vi "Sweep iteration instruction generator (SubVI).vi"(4 "Current iteration":i32, 6 "Angle theta [degrees]":dbl, 7 "Sweep plane & fixed axis":string, 9 "Magnetic field strength [µT]":dbl, 10 "Number of steps":dbl, 11 "Octant":string) -> (0 "Magnetic field z [µT]":dbl, 1 "Magnetic field y [µT]":dbl, 2 "Magnetic field x [µT]":dbl, 3 "Azimuthal angle \"phi\"":dbl, 5 "String: instructions to be sent to PS":string)   [LabVIEW 2018]
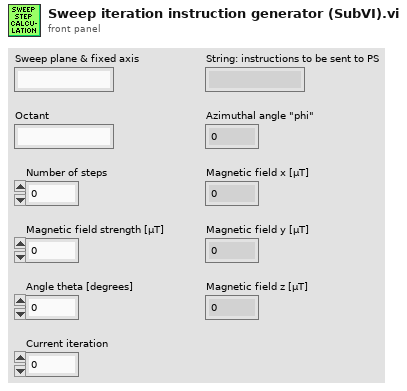
[diagram p1: front panel]
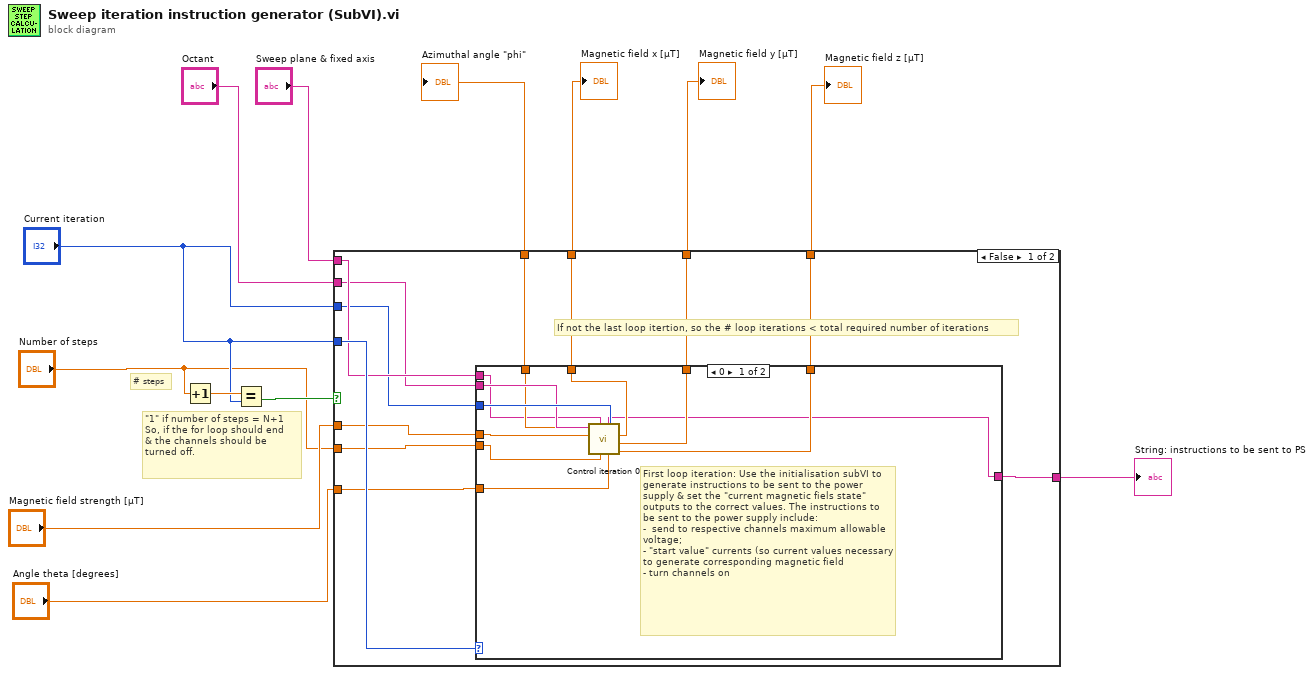
[diagram p0: block diagram]
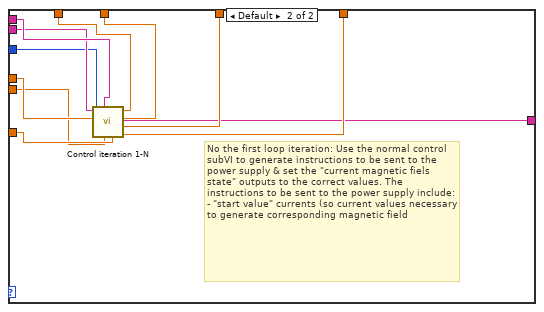
[diagram p2: hidden frame]
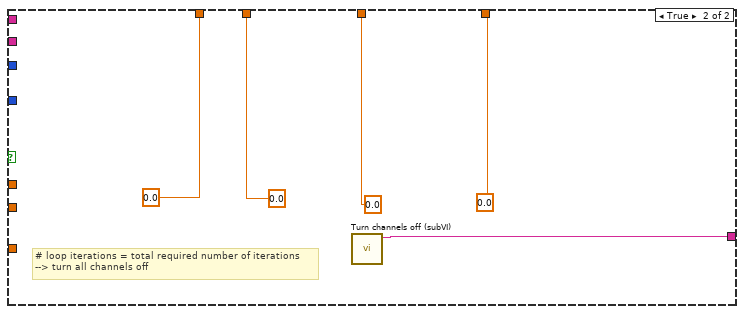
[diagram p3: hidden frame]
diagram:
  # "\"1\" if number of steps = N+1\nSo, if the for loop should end \n& the channels should be \nturned off."
  # "# steps"
  n1 = Increment(x="Number of steps") -> (x+1=w13:dbl)
  n2 = Equal?(x=w13, y="Current iteration") -> (x = y?=w3:bool)
  n3 = case shown="False" w3 {
    tunnel: [w18 0.0 ("Azimuthal angle \"phi\"")] -> w4
    tunnel: [w15 0.0 ("Magnetic field x [µT]")] -> w8
    tunnel: [w17 0.0 ("Magnetic field y [µT]")] -> w9
    tunnel: [w16 0.0 ("Magnetic field z [µT]")] -> w10
    tunnel: "Current iteration" -> [w25 _]
    tunnel: "Sweep plane & fixed axis" -> [w24 _]
    tunnel: "Octant" -> [w23 _]
    tunnel: "Magnetic field strength [µT]" -> [w22 _]
    tunnel: "Current iteration" -> [w21 _]
    tunnel: "Number of steps" -> [w20 _]
    tunnel: "Angle theta [degrees]" -> [w19 _]
    tunnel: [w14 w48] -> w11
    frame False {
      # "If not the last loop itertion, so the # loop iterations < total required number of iterations"
      n4 = case shown="0" w25 {
        tunnel: w24 -> [w27 w47]
        tunnel: w23 -> [w31 w46]
        tunnel: w22 -> [w36 w45]
        tunnel: w21 -> [w35 w38]
        tunnel: w20 -> [w26 w39]
        tunnel: w19 -> [w34 w44]
        tunnel: [w28 w43] -> w18
        tunnel: [w30 w42] -> w15
        tunnel: [w32 w41] -> w17
        tunnel: [w33 w40] -> w16
        tunnel: [w29 w37] -> w14
        frame 0 {
          # "First loop iteration: Use the initialisation subVI to generate instructions to be sent to the power supply & set the \"current magnetic fiels state\" outputs to the correct values. The instructions to be sent to the power supply include:\n-  send to respective channels maximum allowable voltage;\n- \"start value\" currents (so current values necessary to generate corresponding magnetic field \n- turn channels on"
          n5 = call "Control iteration 0.vi"("Angle theta [degrees]"=w34, "Number of steps"=w26, "Sweep plane & fixed axis"=w27, "Current iteration"=w35, "Magnetic field strength [µT]"=w36, "Octant"=w31) -> ("Magnetic field z [µT]"=w33:dbl, "Magnetic field y [µT]"=w32:dbl, "Magnetic field x [µT]"=w30:dbl, "Current angle"=w28:dbl, "Output instructions iteration 0"=w29:string)  [unwired: 1 in]
        }
        frame Default {
          # "No the first loop iteration: Use the normal control subVI to generate instructions to be sent to the power supply & set the \"current magnetic fiels state\" outputs to the correct values. The instructions to be sent to the power supply include:\n- \"start value\" currents (so current values necessary to generate corresponding magnetic field"
          n6 = call "Control iteration 1-N.vi"("Angle theta [degrees]"=w44, "Number of steps"=w39, "Sweep plane & fixed axis"=w47, "Current iteration"=w38, "Magnetic field strength [µT]"=w45, "Octant"=w46) -> ("Magnetic field z [µT]"=w40:dbl, "Magnetic field y [µT]"=w41:dbl, "Magnetic field x [µT]"=w42:dbl, "Current angle"=w43:dbl, "Output instructions 1->N"=w37:string)  [unwired: 1 in]
        }
      }
    }
    frame True {
      # "# loop iterations = total required number of iterations\n--> turn all channels off"
      n7 = call "Turn channels off (subVI).vi"() -> ("String"=w48:string)  [unwired: 11 in]
    }
  }
  "String: instructions to be sent to PS" <- w11
  "Magnetic field z [µT]" <- w10
  "Magnetic field y [µT]" <- w9
  "Magnetic field x [µT]" <- w8
  "Azimuthal angle \"phi\"" <- w4
